vi "Calcul_Nori.vi"(11 "Cale Imagine":path) -> (2 "2D Picture":picture, 3 "Procent Nori":dbl)   [LabVIEW 2024]
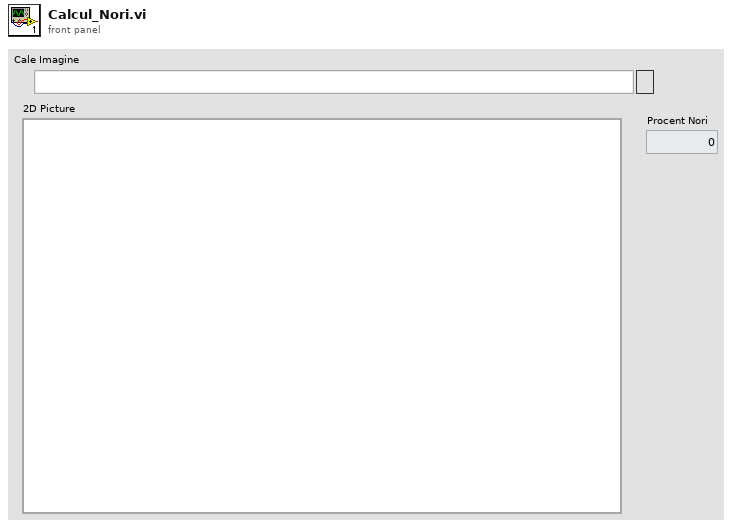
[diagram p1: front panel]
types:
  T1 = typedef "imagedata.ctl" = cluster{"image type":i32, "image depth":i32, "image":u8[], "mask":u8[], "colors":u32[], "Rectangle":cluster{"left":i16, "top":i16, "right":i16, "bottom":i16}}
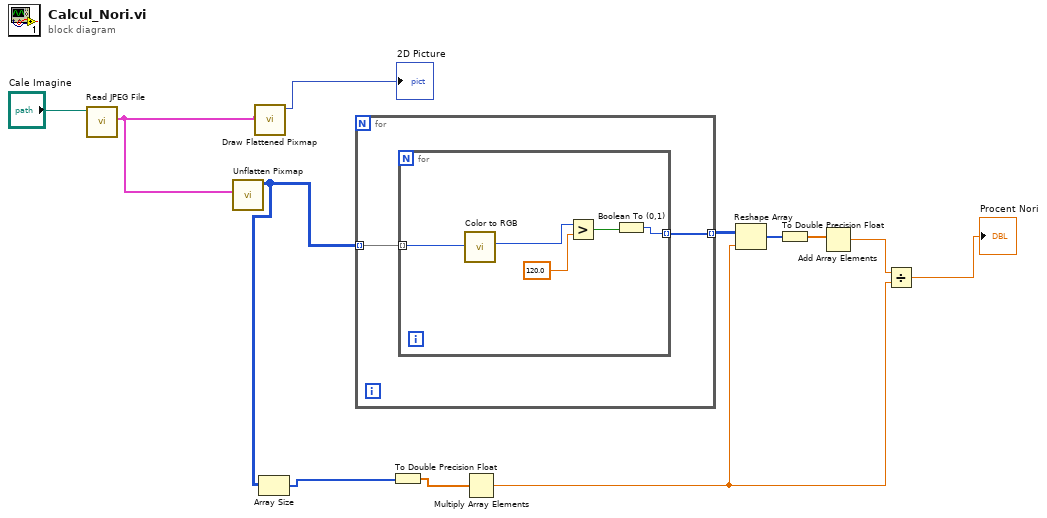
[diagram p0: block diagram]
diagram:
  n1 = call <vilib>:"Read JPEG File.vi"("path to JPEG file"="Cale Imagine") -> ("image data"=w1:T1)  [unwired: 8 in, 2 out]
  n2 = call <vilib>:"Unflatten Pixmap.vi"("image data"=w1) -> ("24-bit pixmap"=w11:u32[][])  [unwired: 4 in, 6 out]
  n3 = call <vilib>:"Draw Flattened Pixmap.vi"("image data"=w1) -> ("new picture"=→"2D Picture":picture)  [unwired: 8 in]
  n4 = Array Size(array=w11) -> (size(s)=w5:i32[])
  n5 = for {
    tunnel: w11 -> [w14] mode=indexing
    tunnel: [w13] -> w10 mode=indexing
    n6 = for {
      tunnel: w14 -> [w19] mode=indexing
      tunnel: [w15] -> w13 mode=indexing
      n7 = call <vilib>:"Color to RGB.vi"("Color"=w19) -> ("R"=w18:u8)  [unwired: 3 out]
      n8 = Greater?(x=w18, y=120.0) -> (0:w16:bool)
      n9 = Boolean To (0,1)(Boolean=w16) -> (0, 1=w15:i16)
    }
  }
  n10 = To Double Precision Float(number=w5) -> (double precision float=w4:dbl[])
  n11 = Multiply Array Elements(1:w4) -> (0:w2:dbl)
  n12 = Reshape Array "Reshape Array"(w10, w2) -> (w6:i16[])
  n13 = To Double Precision Float(number=w6) -> (double precision float=w7:dbl[])
  n14 = Add Array Elements(numeric array=w7) -> (sum=w3:dbl)
  n15 = Divide(x=w3, y=w2) -> (x/y=→"Procent Nori":dbl)
